vi "test_ac_source.vi"() -> ()   [LabVIEW 2020]
uses:
  control_software/Filter function meter/General AC source/Type definitions/AC Source type.ctl
  control_software/Filter function meter/General AC source/Type definitions/AC Source.ctl
panel:
  out "Init status":string
  out "error out":errorcluster
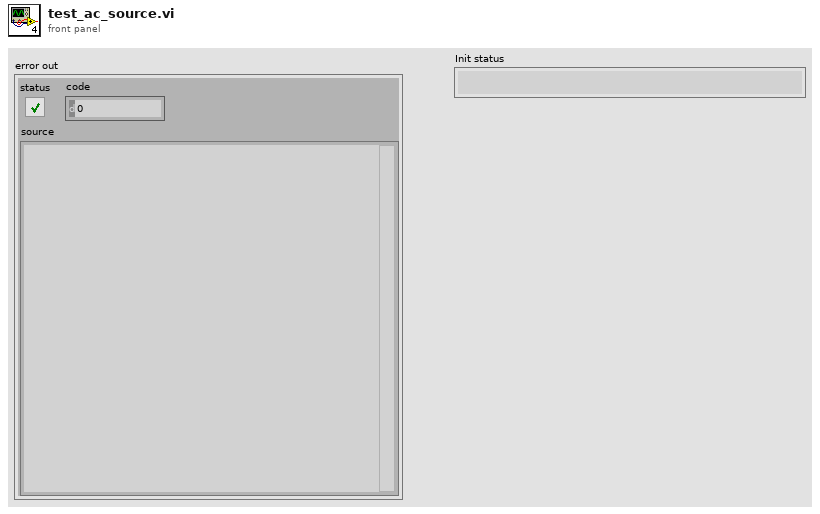
[diagram p1: front panel]
types:
  T1 = typedef "AC Source.ctl" = cluster{"AC Source type":T2, "VISA":refnum<visa-resource-name>, "Ref. clock (Hz)":dbl}
  T2 = typedef "AC Source type.ctl" = enum16{"Fluke 5XXX calibrator", "Tektronix AFG3101C", "dummy"}
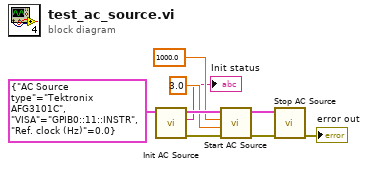
[diagram p0: block diagram]
diagram:
  n1 = call "Init AC Source.vi"("AC source"=T1 {"AC Source type"=enum."Tektronix AFG3101C", "VISA"="GPIB0::11::INSTR", "Ref. clock (Hz)"=0.0}) -> ("error out"=w8:errorcluster, "Init status"=→"Init status":string, "AC source out"=w7:T1)  [unwired: 8 in]
  n2 = call "Start AC Source.vi"("error in (no error)"=w8, "Signal amplitude (V)"=3.0, "Signal frequency  (Hz)"=1000.0, "AC source"=w7) -> ("error out"=w9:errorcluster, "AC source out"=w5:T1)  [unwired: 6 in]
  n3 = call "Stop AC Source.vi"("error in (no error)"=w9, "AC source"=w5) -> ("error out"=→"error out":errorcluster)  [unwired: 8 in, 1 out]
